vi "HDI Pad Group Imaging.vi"() -> ()   [LabVIEW 2011]
uses:
  Shared Components/Config Manager Class/Type Definitions/Part Type.ctl
  Shared Components/CameraTool Class/CameraTool Class.lvclass
  Shared Components/Config Manager Class/Config Manager Class.lvclass
  Shared Components/Gantry Class/Gantry Class.lvclass
panel:
  in  "Config Folder":path=path "C:/Users/Husker/Desktop/gantry/Config"
  out "error out":errorcluster
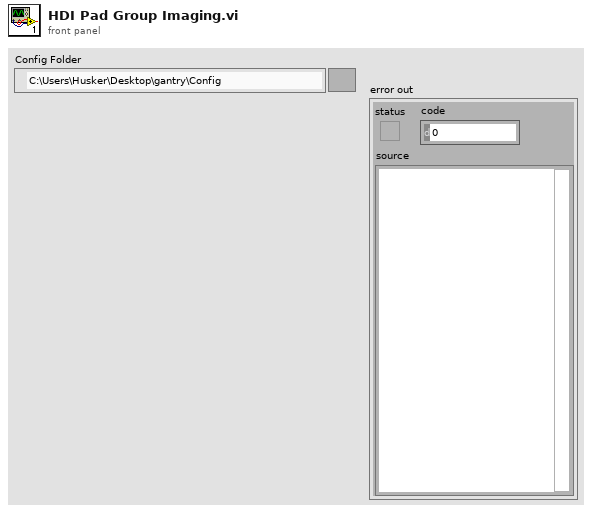
[diagram p1: front panel]
types:
  T1 = typedef "Part Type.ctl" = enum16{"BBM", "HDI", "GLUERESERVOIR", "STAMP", "WEIGHT"}
  T2 = cluster{"Pad Group":i32, "Slot":i32, "Chuck":i32}
  T3 = typedef "Physical Image.ctl" = cluster{"Image Position":refnum<class "Vec3d Class.lvclass">, "Image Reference":T4, "Field of View":cluster{"x(mm)":dbl, "y(mm)":dbl}}
  T4 = typedef "IMAQ Image.ctl" = refnum<image>
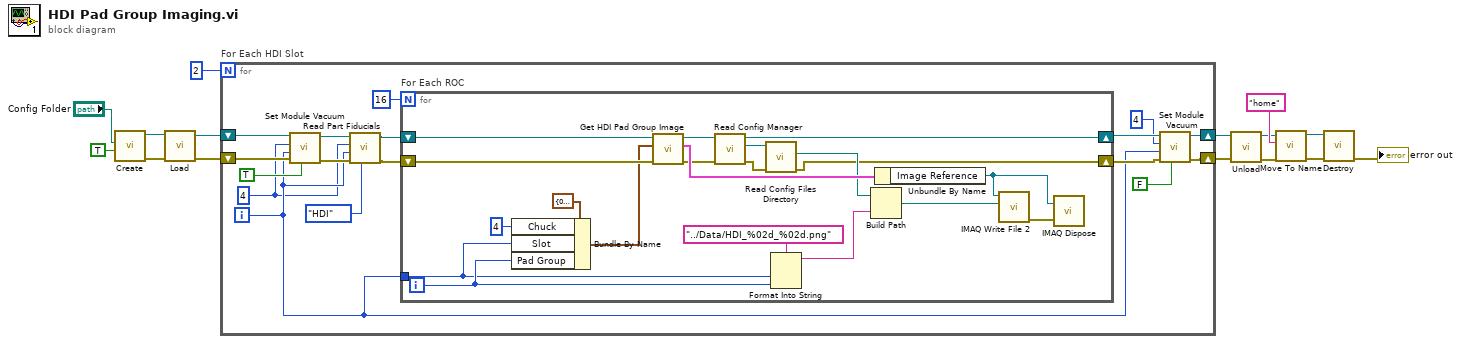
[diagram p0: block diagram]
diagram:
  n1 = call "Create.vi"("HOME?"=TRUE, "Config Folder"="Config Folder") -> ("error out"=w5:errorcluster, "Gantry out"=w6:refnum<class "Gantry Class.lvclass">)  [unwired: 8 in]
  n2 = call "Load.vi"("error in"=w5, "Gantry In"=w6) -> ("error out"=w7:errorcluster, "CameraTool out"=w8:refnum<class "CameraTool Class.lvclass">)  [unwired: 8 in]
  n3 = for "For Each HDI Slot" {
    N: 2 -> [_]
    shift-right: [w28] -> w3
    shift-left: w7 -> [w22]
    shift-right: [w25] -> w4
    shift-left: w8 -> [w24]
    i -> [w17]
    w16 = 4 ("Chuck Number")
    n4 = call-dynamic "Set Module Vacuum.vi"("On/Off"=TRUE, "error in"=w22, "Slot Number"=w17, "Chuck Number"=w16, "Gantry in"=w24) -> ("error out"=w21:errorcluster, "Gantry out"=w23:refnum<class "CameraTool Class.lvclass">)  [unwired: 5 in]
    n5 = call-dynamic "Read Part Fiducials.vi"("Part Type"=Part_Type."HDI", "error in"=w21, "Slot"=w17, "Chuck"=w16, "CameraTool in"=w23) -> ("error out"=w26:errorcluster, "CameraTool out"=w27:refnum<class "CameraTool Class.lvclass">)  [unwired: 4 in, 1 out]
    n6 = for "For Each ROC" {
      N: 16 -> [_]
      shift-right: [w40] -> w30
      shift-left: w27 -> [w48]
      shift-right: [w35] -> w29
      shift-left: w26 -> [w47]
      tunnel: w17 -> [w45]
      i -> [w46]
      n7 = Bundle By Name(cluster=T2 {"Pad Group"=0, "Slot"=0, "Chuck"=0} ("HDI Pad Group"), "Chuck"=4, "Slot"=w45, "Pad Group"=w46) -> (w42:T2)
      n8 = call-dynamic "Get HDI Pad Group Image.vi"("error in"=w47, "HDI Pad Group"=w42, "CameraTool in"=w48) -> ("error out"=w39:errorcluster, "HDI Pad Group Physical Image"=w52:T3, "CameraTool out"=w41:refnum<class "CameraTool Class.lvclass">)  [unwired: 6 in]
      n9 = call-dynamic "Read Config Manager.vi"("error in"=w39, "Gantry in"=w41) -> ("error out"=w37:errorcluster, "Config Manager"=w38:refnum<class "Config Manager Class.lvclass">, "Gantry out"=w40:refnum<class "CameraTool Class.lvclass">)  [unwired: 7 in]
      n10 = call-dynamic "Read Config Files Directory.vi"("error in (no error)"=w37, "Config Manager Class in"=w38) -> ("error out"=w35:errorcluster, "Config Files Directory"=w36:path)  [unwired: 7 in, 1 out]
      n11 = Format Into String(format string="../Data/HDI_%02d_%02d.png" ("name or relative path"), w45, w46) -> (resulting string=w50:string)  [unwired: 2 in, 1 out]
      n12 = Build Path(base path=w36, name or relative path=w50) -> (appended path=w49:path)
      n13 = Unbundle By Name(w52) -> ("Image Reference"=w34:T4)
      n14 = call-poly "IMAQ Write File 2"("File Path"=w49, "Image"=w34) -> ("error out"=w33:errorcluster)  [unwired: 8 in, 1 out]
      n15 = call "IMAQ Dispose"("Image"=w34, "error in (no error)"=w33) -> ()  [unwired: 4 in, 1 out]
    }
    n16 = call-dynamic "Set Module Vacuum.vi"("On/Off"=FALSE, "error in"=w29, "Slot Number"=w17, "Chuck Number"=4, "Gantry in"=w30) -> ("error out"=w28:errorcluster, "Gantry out"=w25:refnum<class "CameraTool Class.lvclass">)  [unwired: 5 in]
  }
  n17 = call "Unload.vi"("error in"=w3, "CameraTool in"=w4) -> ("error out"=w1:errorcluster, "Gantry out"=w2:refnum<class "Gantry Class.lvclass">)  [unwired: 8 in]
  n18 = call-dynamic "Move To Name.vi"("error in"=w1, "Destination Name"="home", "Gantry in"=w2) -> ("error out"=w10:errorcluster, "Gantry out"=w11:refnum<class "Gantry Class.lvclass">)  [unwired: 7 in]
  n19 = call "Destroy.vi"("error in"=w10, "Gantry Class in"=w11) -> ("error out"=→"error out":errorcluster)  [unwired: 9 in]
